vi "DrawItemsStatic.vi"(8 "error in (no error)":errorcluster, 11 "OrderSelection in":refnum<class "OrderSelection.lvclass">) -> (0 "error out":errorcluster, 3 "OrderSelection out":refnum<class "OrderSelection.lvclass">)   [LabVIEW 2020, in "OrderSelection.lvclass"]
uses:
  OrderSelection.lvclass
  OrderSelection.lvclass/OrderSelection.ctl
  Read Items.vi
  Read ItemGraphic.vi
  Read SelectedItem.vi
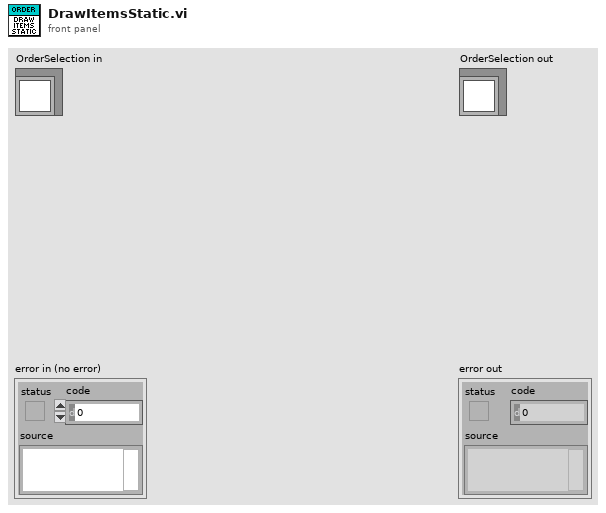
[diagram p1: front panel]
types:
  T1 = cluster{"horizontal":enum16{"left", "center", "right"}, "vertical":enum16{"top", "center", "bottom"}}
  T2 = cluster{"Horizontal Shift":i16, "Vertical Shift":i16}
  T3 = cluster{"Width":i16, "Style":enum32{"Solid", "Dash", "Dot", "DashDot", "DashDotDot"}}
  T4 = cluster{"left":i16, "top":i16, "right":i16, "bottom":i16}
  T5 = typedef "imagedata.ctl" = cluster{"image type":i32, "image depth":i32, "image":u8[], "mask":u8[], "colors":u32[], "Rectangle":cluster{"left":i16, "top":i16, "right":i16, "bottom":i16}}
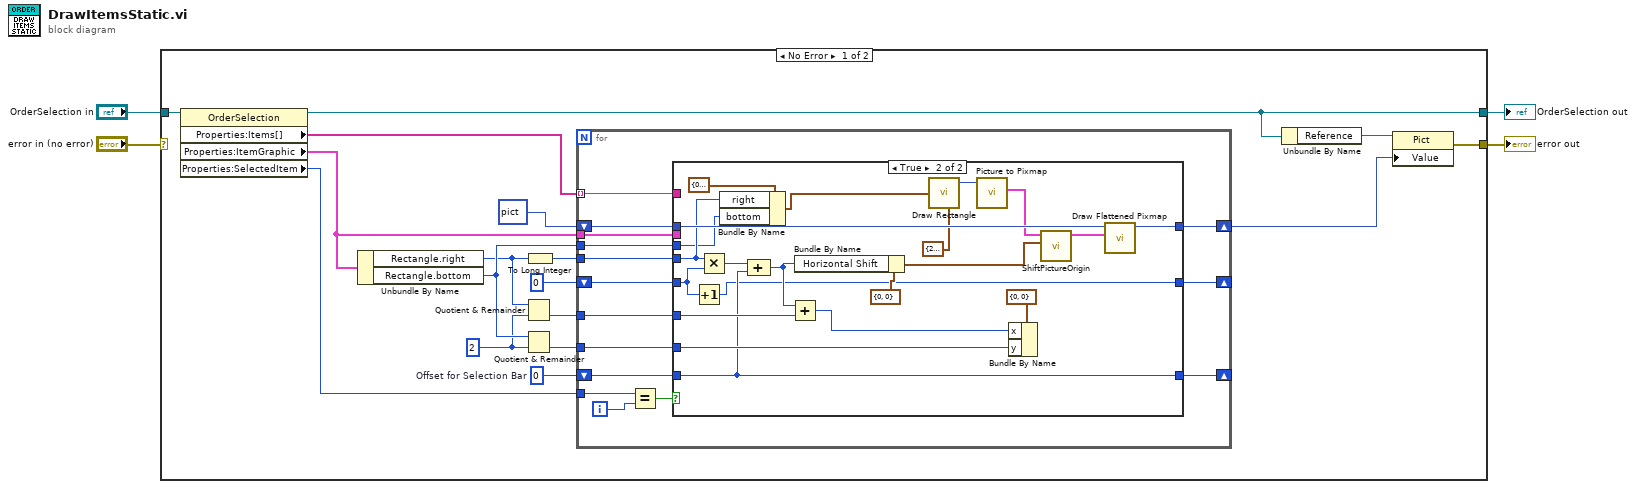
[diagram p0: block diagram]
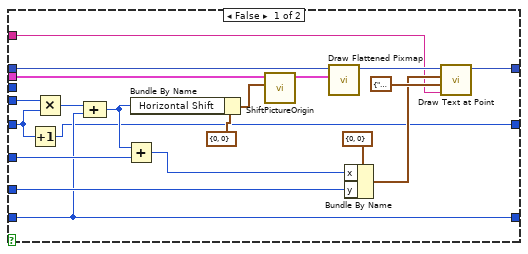
[diagram p2: hidden frame]
diagram:
  n1 = case shown="No Error" "error in (no error)" {
    selector: "error in (no error)" -> [_ w79]
    tunnel: [w6 w79] -> w3
    tunnel: [w7 w78] -> w1
    tunnel: "OrderSelection in" -> [w8 w78]
    frame No Error {
      w19 = 0  # Offset for Selection Bar
      w12 = i16 2 ("y")
      n2 = property class="OrderSelection"(reference=w8) -> (reference out=w7:refnum<class "OrderSelection.lvclass">, "Properties:Items[]"=w17:string[], "Properties:ItemGraphic"=w18:T5, "Properties:SelectedItem"=w5:i32)  [unwired: 1 in, 1 out]
      n3 = Unbundle By Name(w18) -> ("Rectangle.right"=w11:i16, "Rectangle.bottom"=w21:i16)
      n4 = Quotient & Remainder(x=w11, y=w12) -> (floor(x/y)=w13:i16)  [unwired: 1 out]
      n5 = Quotient & Remainder(x=w21, y=w12) -> (floor(x/y)=w14:i16)  [unwired: 1 out]
      n6 = To Long Integer(number=w11) -> (32bit integer=w10:i32)
      n7 = for {
        tunnel: w18 -> [w36]
        shift-right: [w33] -> w16
        shift-left: picture data[5B] ("new picture") -> [w35]
        tunnel: w10 -> [w34]
        tunnel: w13 -> [w31]
        tunnel: w14 -> [w32]
        tunnel: w17 -> [w30] mode=indexing
        tunnel: w5 -> [w29]
        shift-right: [w26] -> _
        shift-left: w19 -> [w27]
        shift-right: [w23] -> _
        shift-left: 0 -> [w24]
        tunnel: w21 -> [w22]
        i -> [w25]
        n8 = Equal?(x=w29, y=w25) -> (x = y?=w28:bool)
        n9 = case shown="True" w28 {
          tunnel: w36 -> [w54 _]
          tunnel: w35 -> [w51 w75]
          tunnel: w34 -> [w50 w61]
          tunnel: [w49 w77] -> w33
          tunnel: w32 -> [w40 w69]
          tunnel: w31 -> [w45 w73]
          tunnel: w30 -> [w43 _]
          tunnel: w27 -> [w39 w68]
          tunnel: [w39 w68] -> w26
          tunnel: w24 -> [w37 w66]
          tunnel: [w38 w67] -> w23
          tunnel: w22 -> [_ w60]
          frame False {
            n10 = Increment(x=w37) -> (x+1=w38:i32)
            n11 = Multiply(x=w50, y=w37) -> (x*y=w42:i32)
            n12 = Compound Arithmetic op=ADD(w42, w39) -> (w41:i32)
            n13 = Add(x=w41, y=w45) -> (x+y=w44:i32)
            n14 = Bundle By Name(cluster=T2 {"Horizontal Shift"=0, "Vertical Shift"=0} ("Shift(0, 0)"), "Horizontal Shift"=w41) -> (w52:T2)
            n15 = call "ShiftPictureOrigin.vi"("Shift(0, 0)"=w52, "image data IN"=w54) -> ("image data OUT"=w56:T5)  [unwired: 8 in, 1 out]
            n16 = call <vilib>:"Draw Flattened Pixmap.vi"("image data"=w56, "picture"=w51) -> ("new picture"=w55:picture)  [unwired: 7 in]
            n17 = Bundle By Name(cluster=cluster{"x":i16, "y":i16} {"x"=0, "y"=0} ("origin"), "x"=w44, "y"=w40) -> (w46:cluster{"x":i16, "y":i16})
            n18 = call <vilib>:"Draw Text at Point.vi"("text"=w43, "alignment(left, top)"=T1 {"horizontal"=enum."center", "vertical"=enum."center"}, "origin"=w46, "picture"=w55) -> ("new picture"=w49:picture)  [unwired: 6 in, 1 out]
          }
          frame True {
            n19 = Increment(x=w66) -> (x+1=w67:i32)
            n20 = Multiply(x=w61, y=w66) -> (x*y=w71:i32)
            n21 = Bundle By Name(cluster=T4 {"left"=0, "top"=0, "right"=0, "bottom"=0} ("rect"), "right"=w61, "bottom"=w60) -> (w58:T4)
            n22 = Compound Arithmetic op=ADD(w71, w68) -> (w70:i32)
            n23 = Add(x=w70, y=w73) -> (x+y=w72:i32)
            n24 = Bundle By Name(cluster=T2 {"Horizontal Shift"=0, "Vertical Shift"=0} ("Shift(0, 0)"), "Horizontal Shift"=w70) -> (w64:T2)
            n25 = call <vilib>:"Draw Rectangle.vi"("rect"=w58, "pen"=T3 {"Width"=2, "Style"=enum."Dot"}) -> ("new picture"=w57:picture)  [unwired: 7 in]
            n26 = call <vilib>:"Picture to Pixmap.vi"("picture"=w57) -> ("image data"=w63:T5)  [unwired: 9 in, 1 out]
            n27 = Bundle By Name(cluster=cluster{"x":i16, "y":i16} {"x"=0, "y"=0} ("origin"), "x"=w72, "y"=w69) -> ()  [unwired: 1 out]
            n28 = call "ShiftPictureOrigin.vi"("Shift(0, 0)"=w64, "image data IN"=w63) -> ("image data OUT"=w65:T5)  [unwired: 8 in, 1 out]
            n29 = call <vilib>:"Draw Flattened Pixmap.vi"("image data"=w65, "picture"=w75) -> ("new picture"=w77:picture)  [unwired: 7 in]
          }
        }
      }
      n30 = Unbundle By Name(w7) -> ("Reference"=w15:refnum<vi>)
      n31 = property class="Pict"(reference=w15, "Value"=w16) -> (error out=w6:errorcluster)  [unwired: 1 in, 1 out]
    }
    frame Error {
    }
  }
  "error out" <- w3
  "OrderSelection out" <- w1
